vi "Receive Menu Selection Event.vi"(8 "error in (no error)":errorcluster, 10 "MenuSelectionMsg":refnum<class "MenuSelectionMsg.lvclass">, 11 "ConcreteViewModel in":refnum<class "ConcreteViewModel.lvclass">) -> (0 "error out":errorcluster, 3 "ConcreteViewModel out":refnum<class "ConcreteViewModel.lvclass">)   [LabVIEW 2015, in "TopLevelApplication.lvlib" / "ConcreteViewModel.lvclass"]
doc: "<License>\nCopyright © 2017 Composed Systems, LLC | All rights reserved\nwww.composed.io\n\nAuthor: Ethan Stern <ethan.stern@composed.io>\n\nThis software is provided \"AS IS\" WITHOUT WARRANTIES, either express or implied, AND IS FOR EDUCATIONAL PURPOSES ONLY.\n</License>"
uses:
  ConcreteViewModel.lvclass
  Framework/ActorEvents/IEventAggregator Messages/MenuSelectionMsg/MenuSelectionMsg.lvclass
  Framework/ActorEvents/IEventAggregator Messages/MenuSelectionMsg/MenuSelectionMsg.lvclass/MenuSelectionMsg.ctl
  Framework/IViewModel/IViewModel/IViewModel.lvclass/IViewModel.ctl
  <vilib>/ActorFramework/Message Enqueuer/Message Enqueuer.lvclass/Message Enqueuer.ctl
  <vilib>/ActorFramework/Message Enqueuer/Enqueue.vi
  <vilib>/ActorFramework/Message Priority Queue/Priority Enqueue.vi
  Framework/IMediator/IMediator Messages/Monitor Msg/Open Bus Monitor Msg.lvclass
  DialogBox/OneButtonDialogBox/OneButtonDialogBox.lvclass
  Framework/IViewModel/IViewModel/IViewModel.lvclass
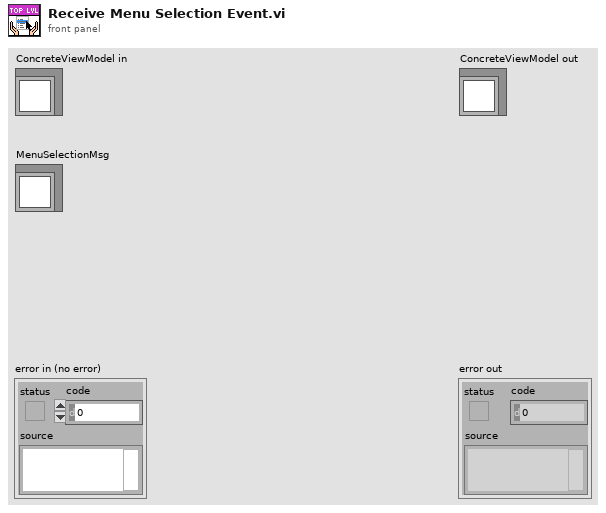
[diagram p1: front panel]
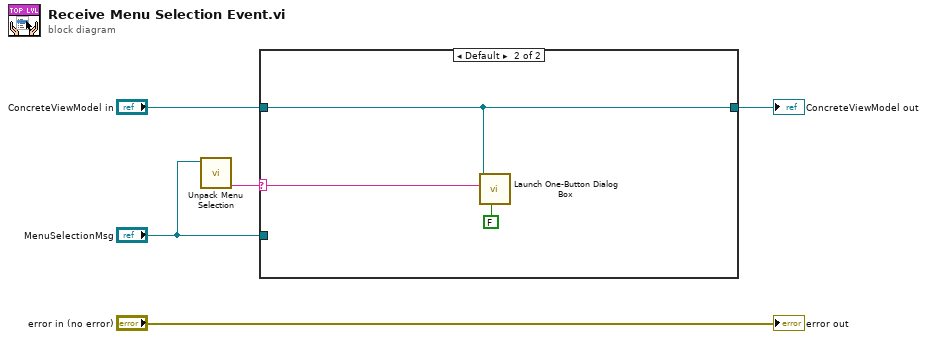
[diagram p0: block diagram]
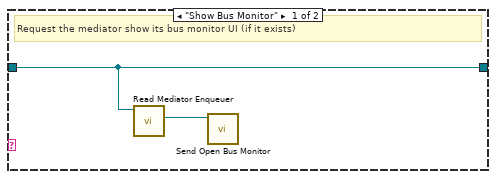
[diagram p2: hidden frame]
diagram:
  n1 = call "Unpack Menu Selection.vi"("MenuSelectionMsg"="MenuSelectionMsg") -> ("Item Tag"=w1:string)  [unwired: 5 in, 5 out]
  n2 = case shown="Default" w1 {
    selector: w1 -> [_ w8]
    tunnel: "MenuSelectionMsg" -> [_ _]
    tunnel: "ConcreteViewModel in" -> [w7 w9]
    tunnel: [w7 w9] -> w3
    frame "Show Bus Monitor" {
      # "Request the mediator show its bus monitor UI (if it exists)"
      n3 = call "Read Mediator Enqueuer.vi"("IViewModel In"=w7) -> ("Mediator Enququer"=w6:refnum<class "Message Enqueuer.lvclass">)  [unwired: 10 in]
      n4 = call "Send Open Bus Monitor.vi"("Message Enqueuer"=w6) -> ()  [unwired: 9 in, 2 out]
    }
    frame Default {
      n5 = call "Launch One-Button Dialog Box.vi"("Modal? (T)"=FALSE, "Message Text"=w8, "Dialog Launcher"=w9) -> ()  [unwired: 8 in, 1 out]
    }
  }
  "ConcreteViewModel out" <- w3
  "error out" <- "error in (no error)"
